vi "LSI218Data_terminate.vi"(8 "error in (no error)":errorcluster, 11 "LSI218Data in":refnum<class "LSI218Data.lvclass">) -> (0 "error out":errorcluster, 3 "LSI218Data out":refnum<class "LSI218Data.lvclass">)   [LabVIEW 2017, in "LSI218Data.lvclass"]
uses:
  LSI218Data.lvclass
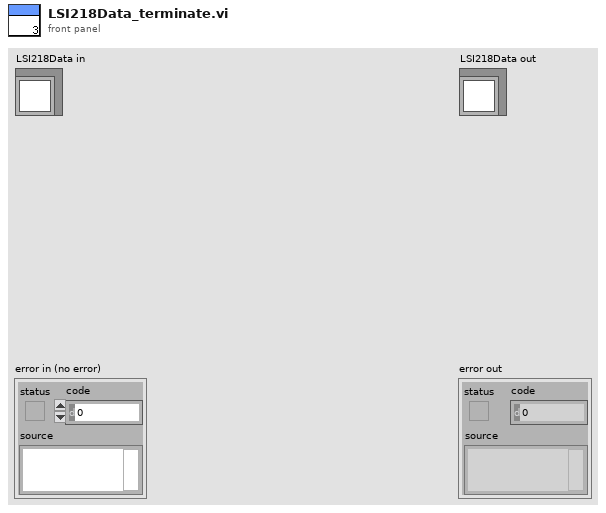
[diagram p1: front panel]
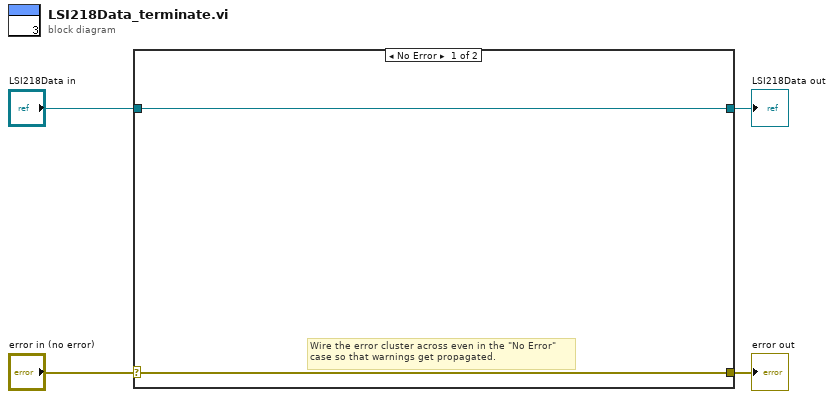
[diagram p0: block diagram]
diagram:
  n1 = case shown="No Error" "error in (no error)" {
    selector: "error in (no error)" -> [w5 w8]
    tunnel: [w5 w8] -> w3
    tunnel: [w6 w7] -> w1
    tunnel: "LSI218Data in" -> [w6 w7]
    frame No Error {
      # "Wire the error cluster across even in the \"No Error\"\ncase so that warnings get propagated."
    }
    frame Error {
    }
  }
  "error out" <- w3
  "LSI218Data out" <- w1
